vi "main_queue_assistant.vi"(0 "queue_type (def=all)":T3=enum."entities_incoming", 1 "action (enq_behind = def)":T8=enum."enq_behind", 2 "entity":T6, 3 "entities":T6[](array[typedef]), 4 "classpath / id (in)":string, 5 "error in (no error)":errorcluster, 6 "classpaths_for_queue_identification (ids)":string[](array[string]), 7 "timestep":dbl, 9 "response":T4) -> (15 "refs (out)":T1, 18 "queues_empty_status (out)":T2[](array[typedef]), 19 "error out":errorcluster)   [LabVIEW 2016]
uses:
  controls/queue_assistant_actions.ctl
  controls/entity.ctl
  controls/entity_type.ctl
  controls/queue_type.ctl
  controls/response.ctl
  controls/response_type.ctl
  controls/queue_status.ctl
  controls/queue_references.ctl
  controls/queue_assistant_runtime_object.ctl
panel:
  in  "queue out":refnum<queue>
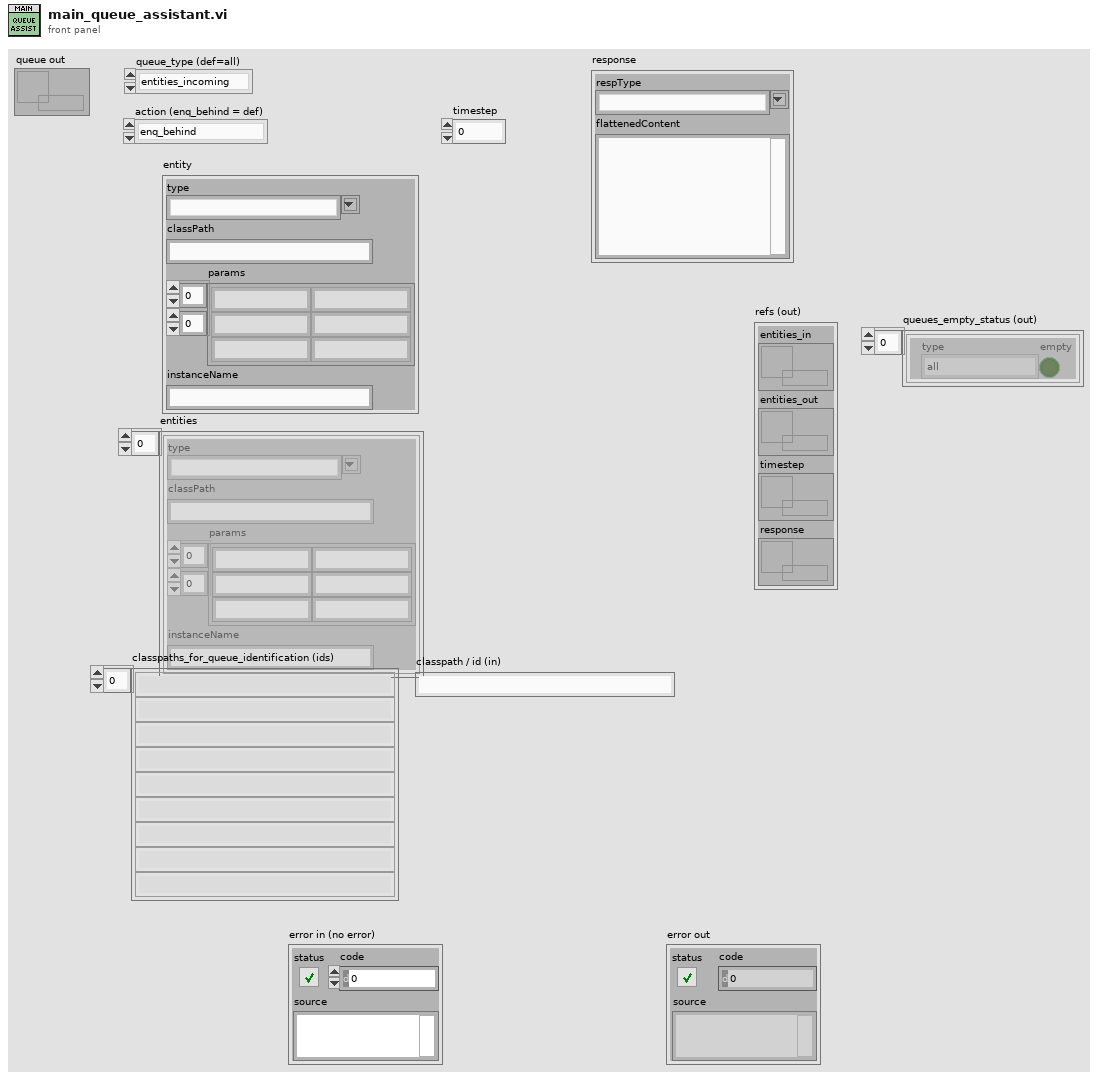
[diagram p1: front panel]
types:
  T1 = typedef "queue_references.ctl" = cluster{"entities_in":refnum<queue>, "entities_out":refnum<queue>, "timestep":refnum<queue>, "response":refnum<queue>}
  T2 = typedef "queue_status.ctl" = cluster{"type":T3, "empty":bool}
  T3 = typedef "queue_type.ctl" = enum16{"all", "dostep", "entities_incoming", "entities_outoing", "response"}
  T4 = typedef "response.ctl" = cluster{"respType":T5, "flattenedContent":string}
  T5 = typedef "response_type.ctl" = string
  T6 = typedef "entity.ctl" = cluster{"type":T7, "classPath":string, "params":string[][], "instanceName":string}
  T7 = typedef "entity_type.ctl" = string
  T8 = typedef "queue_assistant_actions.ctl" = enum16{"--- unused ---", "bulk_enq_ahead", "bulk_enq_behind", "destroy", "empty?", "enq_ahead", "enq_behind", "flush", "get_queues", "init"}
  T9 = typedef "queue_assistant_runtime_object.ctl" = cluster{"classpath":string, "queue":refnum<queue>}
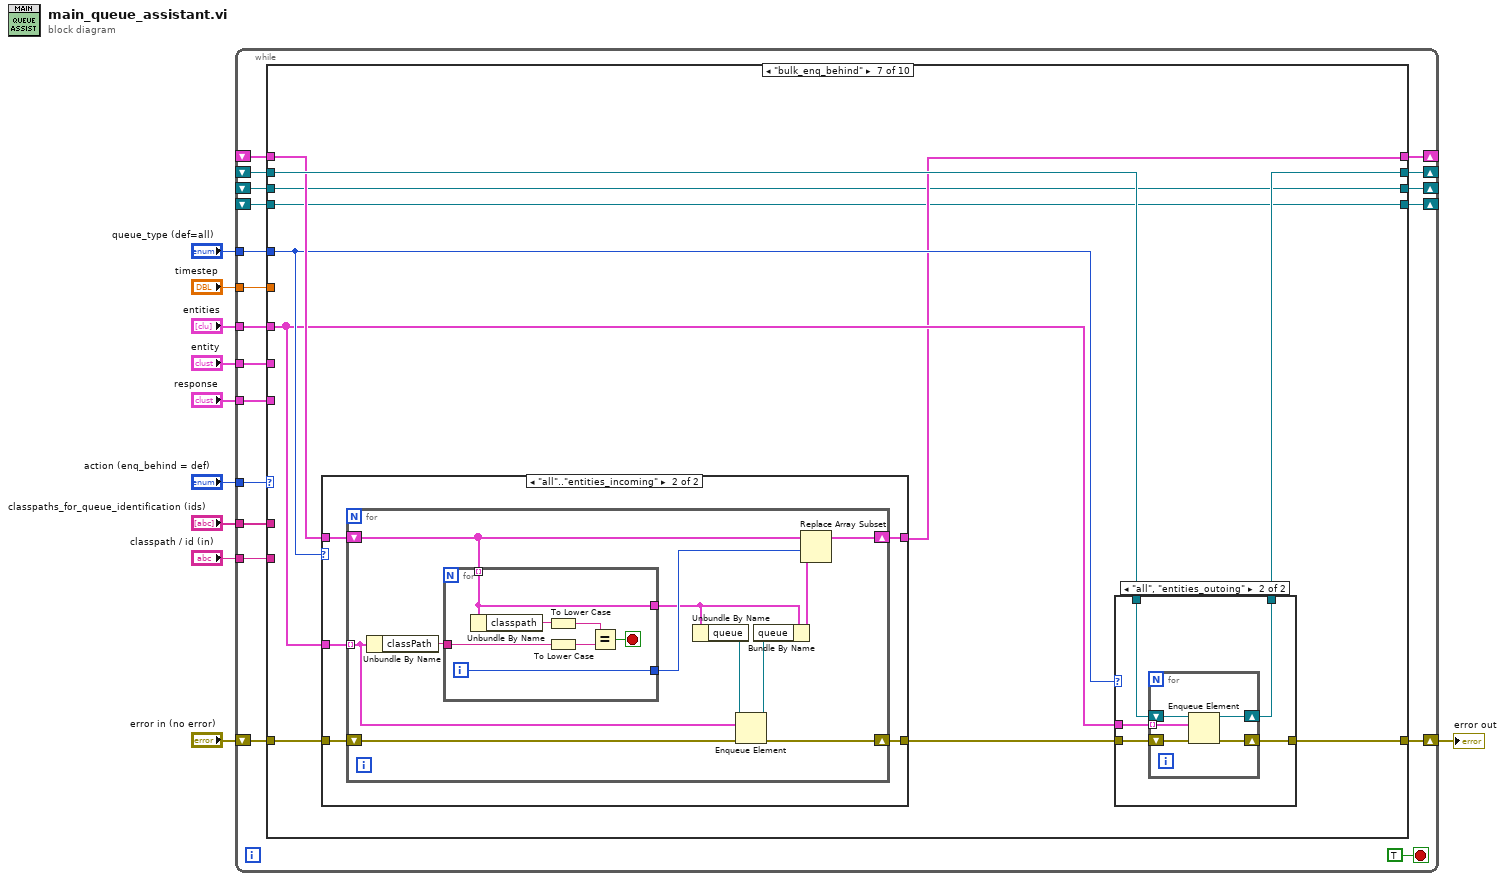
[diagram p0: block diagram]
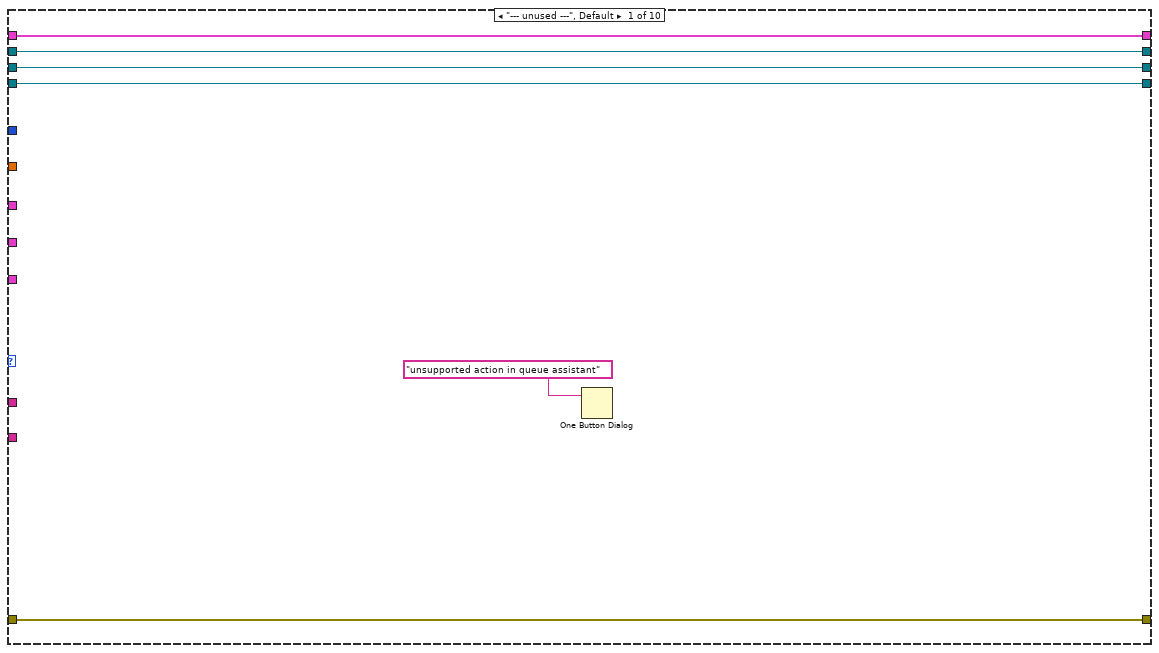
[diagram p2: hidden frame]
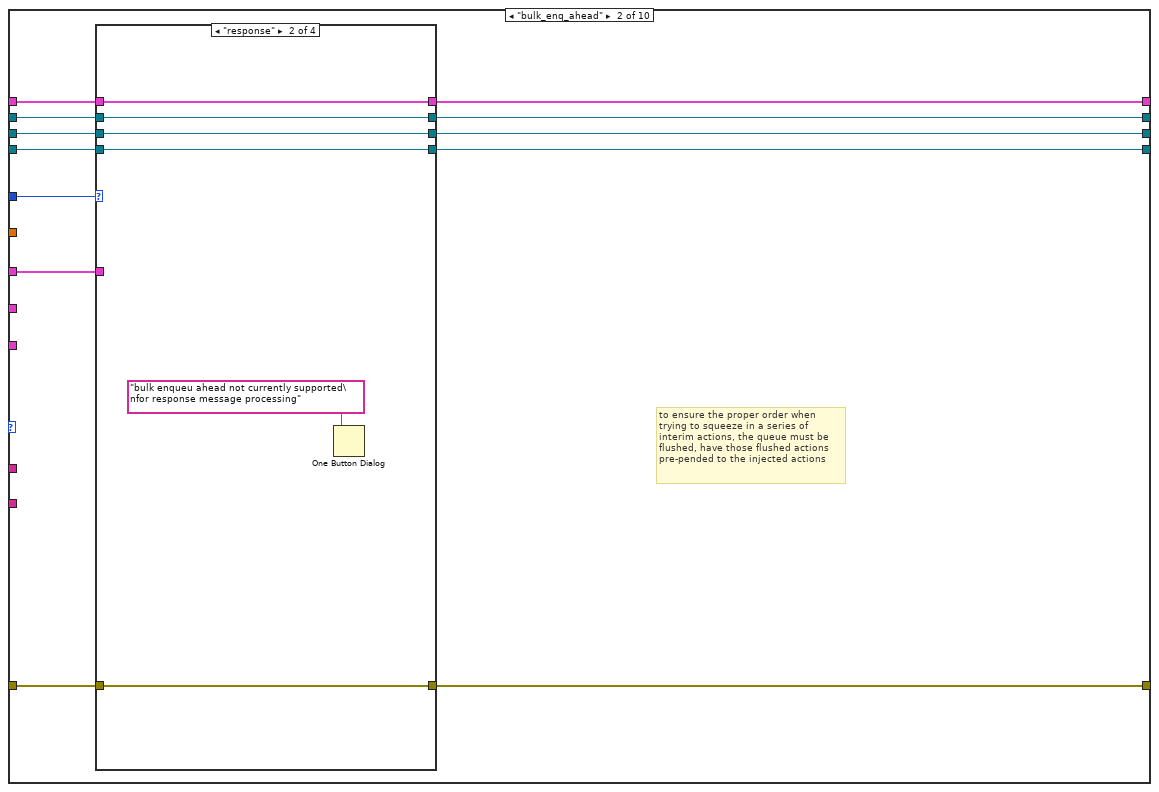
[diagram p3: hidden frame]
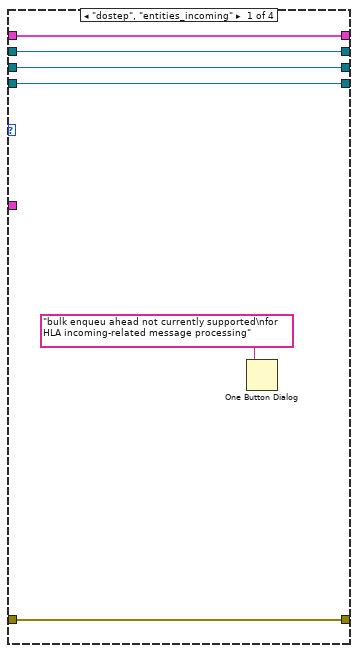
[diagram p4: hidden frame]
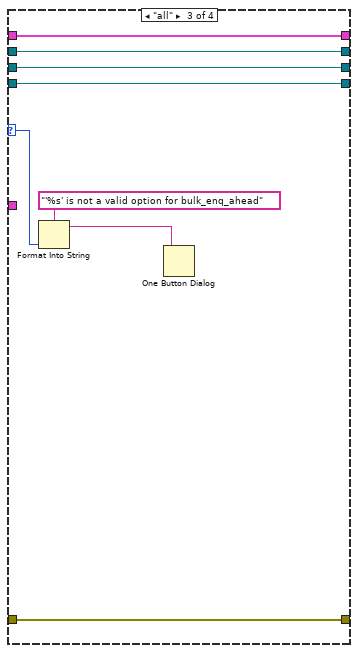
[diagram p5: hidden frame]
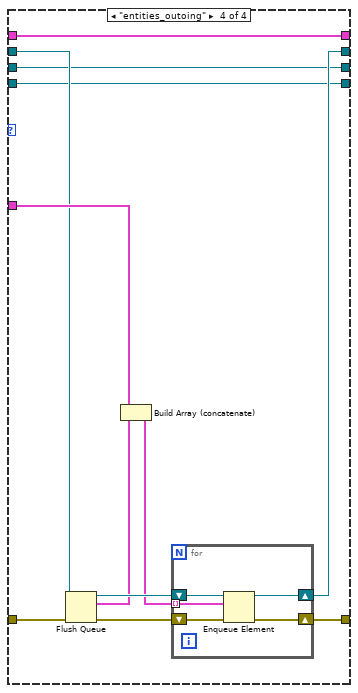
[diagram p6: hidden frame]
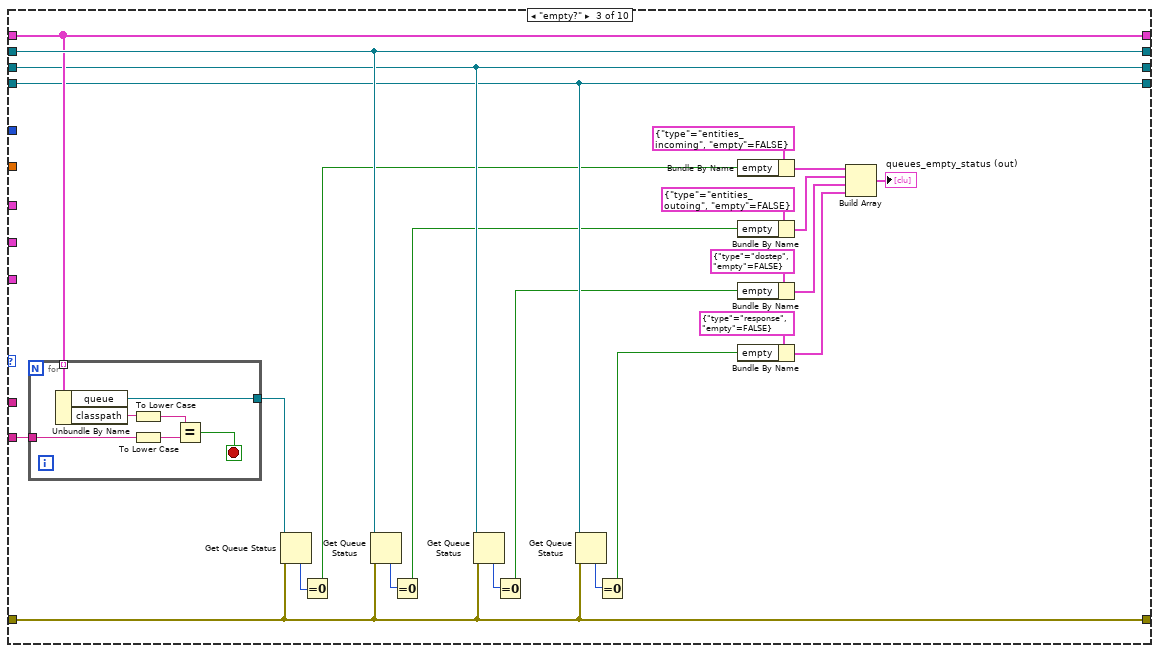
[diagram p7: hidden frame]
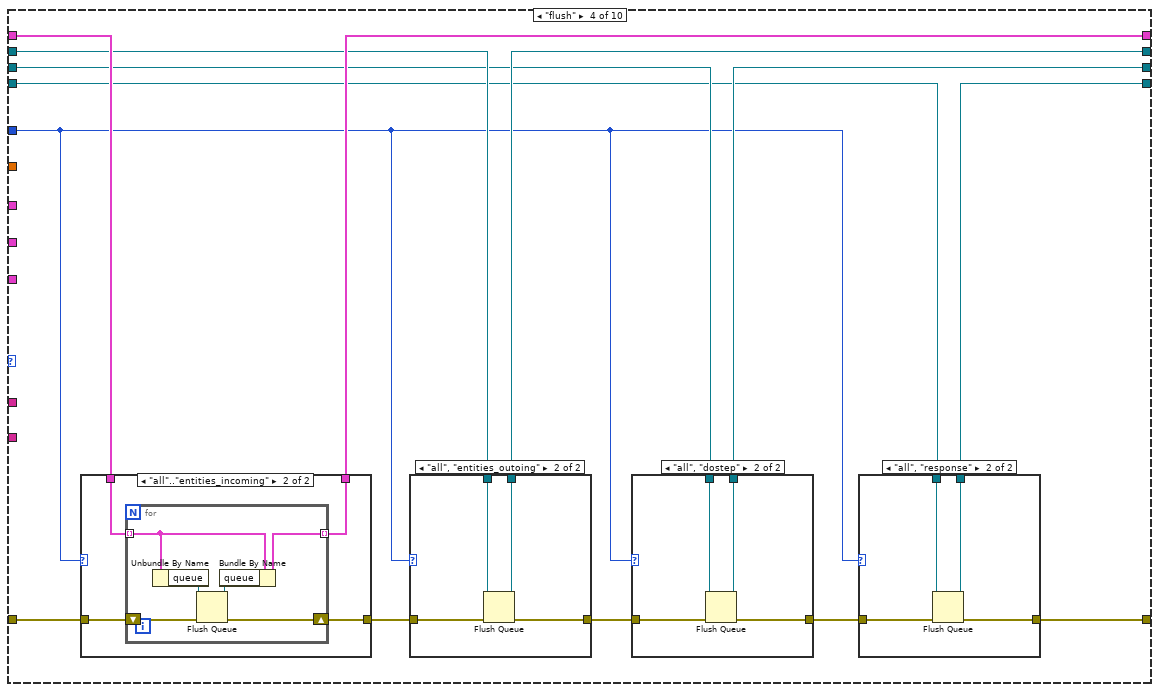
[diagram p8: hidden frame]
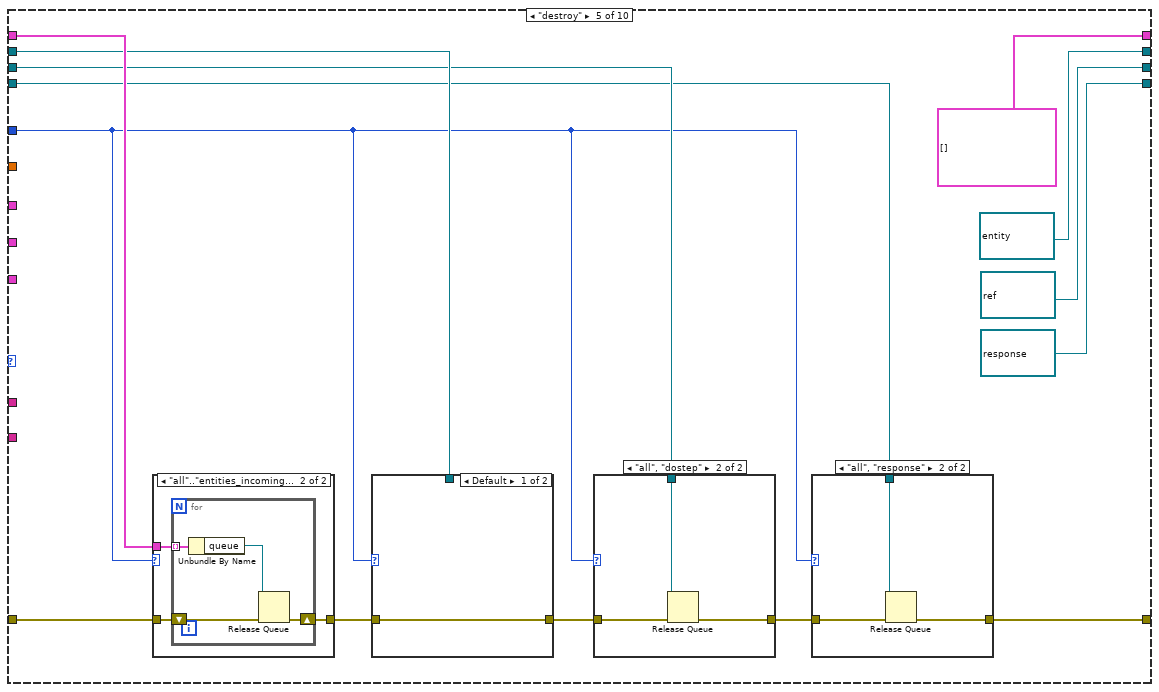
[diagram p13: hidden frame]
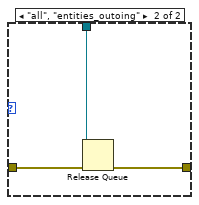
[diagram p16: hidden frame]
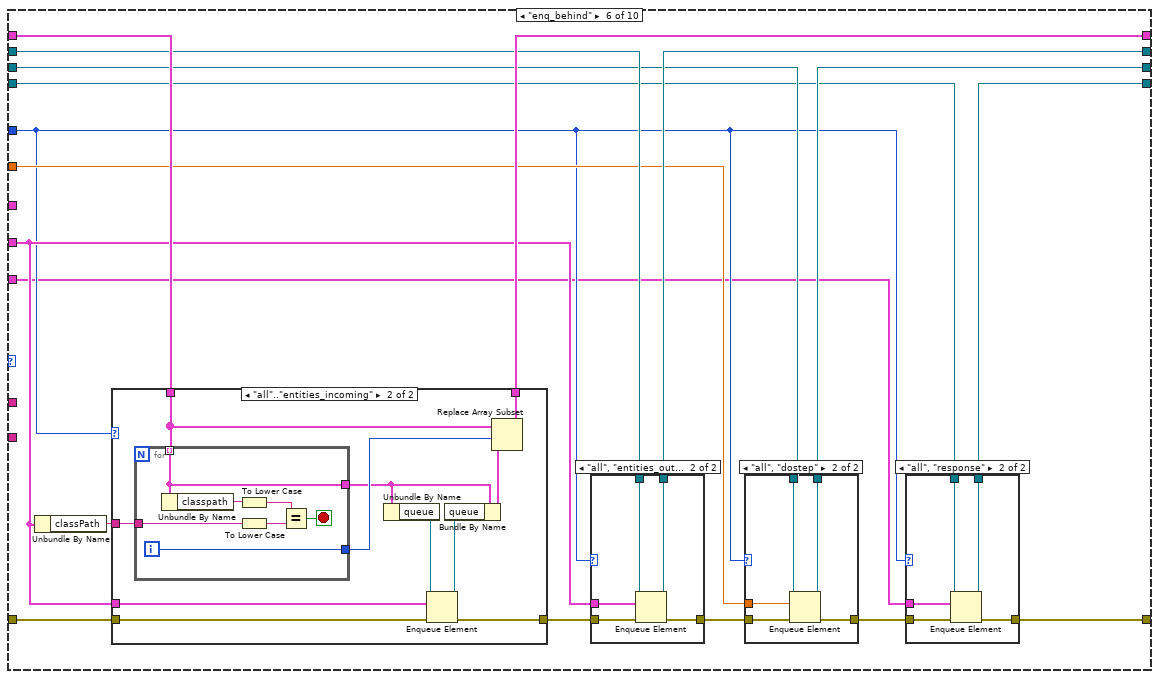
[diagram p18: hidden frame]
diagram:
  n1 = while {
    shift-right: [w22] -> _
    shift-left: _ -> [w25]
    tunnel: "action (enq_behind = def)" -> [w28]
    shift-right: [w26] -> w8
    shift-left: "error in (no error)" -> [w27]
    tunnel: "entity" -> [w24]
    tunnel: "entities" -> [w23]
    shift-right: [w21] -> _
    shift-left: _ -> [w20]
    tunnel: "queue_type (def=all)" -> [w19]
    tunnel: "classpaths_for_queue_identification (ids)" -> [w18]
    tunnel: "classpath / id (in)" -> [w17]
    shift-right: [w15] -> _
    shift-left: _ -> [w16]
    tunnel: "timestep" -> [w14]
    tunnel: "response" -> [w13]
    shift-right: [w12] -> _
    shift-left: _ -> [w11]
    stop <- TRUE stop-if-true
    n2 = case shown="\"bulk_enq_behind\"" w28 {
      tunnel: w27 -> [w34 w47 w85 w128 w173 w210 w257 w315 w366 w392]
      tunnel: [w34 w45 w85 w118 w160 w194 w263 w304 w366 w377] -> w26
      tunnel: w25 -> [w33 w46 w104 w129 w171 w211 w260 w313 w368 _]
      tunnel: w24 -> [_ _ _ _ _ w205 _ w314 _ _]
      tunnel: w23 -> [_ w44 _ _ _ _ w258 _ _ _]
      tunnel: [w33 w42 w104 w127 T9[] [] w209 w256 w312 w368 w391] -> w22
      tunnel: [w32 w40 w106 w124 refnum<queue> refnum ("queue out") w206 w261 w317 w362 w388] -> w21
      tunnel: w20 -> [w32 w41 w106 w125 w170 w207 w262 w318 w362 w389]
      tunnel: w19 -> [_ w43 _ w120 w163 w198 w259 w303 _ _]
      tunnel: w18 -> [_ _ _ _ _ _ _ _ _ w386]
      tunnel: w17 -> [_ _ w105 _ _ _ _ _ w369 _]
      tunnel: w16 -> [w31 w39 w101 w122 w167 w202 w254 w308 w363 w382]
      tunnel: [w31 w38 w101 w121 refnum<queue> refnum ("queue out") w201 w254 w307 w363 w383] -> w15
      tunnel: w14 -> [_ _ _ _ _ w200 _ w309 _ _]
      tunnel: w13 -> [_ _ _ _ _ w197 _ w305 _ _]
      tunnel: [w30 w36 w99 w116 refnum<queue> refnum ("queue out") w195 w253 w301 w364 w379] -> w12
      tunnel: w11 -> [w30 w37 w99 w117 w161 w196 w253 w302 w364 w378]
      frame "--- unused ---", Default {
        n3 = One Button Dialog(message="unsupported action in queue assistant") -> ()  [unwired: 1 in, 1 out]
      }
      frame "bulk_enq_ahead" {
        # "to ensure the proper order when\ntrying to squeeze in a series of\ninterim actions, the queue must be\nflushed, have those flushed actions\npre-pended to the injected actions"
        n4 = case shown="\"response\"" w43 {
          selector: w43 -> [_ _ w63 _]
          tunnel: w47 -> [w51 w57 w65 w79]
          tunnel: w46 -> [w53 w59 w67 w70]
          tunnel: [w51 w57 w65 w77] -> w45
          tunnel: w44 -> [_ _ _ w73]
          tunnel: [w53 w59 w67 w70] -> w42
          tunnel: w41 -> [w52 w58 w66 w72]
          tunnel: [w52 w58 w66 w71] -> w40
          tunnel: [w49 w55 w61 w69] -> w38
          tunnel: w39 -> [w49 w55 w61 w69]
          tunnel: [w48 w54 w60 w68] -> w36
          tunnel: w37 -> [w48 w54 w60 w68]
          frame "dostep", "entities_incoming" {
            n5 = One Button Dialog(message="bulk enqueu ahead not currently supported\nfor HLA incoming-related message processing") -> ()  [unwired: 1 in, 1 out]
          }
          frame "response" {
            n6 = One Button Dialog(message="bulk enqueu ahead not currently supported\nfor response message processing") -> ()  [unwired: 1 in, 1 out]
          }
          frame "all" {
            n7 = Format Into String(format string="'%s' is not a valid option for bulk_enq_ahead", w63) -> (resulting string=w62:string)  [unwired: 2 in, 1 out]
            n8 = One Button Dialog(message=w62) -> ()  [unwired: 1 in, 1 out]
          }
          frame "entities_outoing" {
            n9 = Flush Queue(queue=w72, error in (no error)=w79) -> (queue out=w76:refnum<queue>, remaining elements=w74:T6[], error out=w78:errorcluster)
            n10 = Build Array (concatenate)(w73, w74) -> (w75:T6[])
            n11 = for {
              shift-right: [w83] -> w77
              shift-left: w78 -> [w84]
              shift-right: [w81] -> w71
              shift-left: w76 -> [w82]
              tunnel: w75 -> [w80] mode=indexing
              n12 = Enqueue Element(queue=w82, element=w80, error in (no error)=w84) -> (queue out=w81:refnum<queue>, error out=w83:errorcluster)  [unwired: 1 in, 1 out]
            }
          }
        }
      }
      frame "empty?" {
        n13 = for {
          tunnel: w105 -> [w114]
          tunnel: w104 -> [w110] mode=indexing
          tunnel: [w109] -> w103
          stop <- w111 stop-if-true
          n14 = Unbundle By Name(w110) -> ("queue"=w109:refnum<queue>, "classpath"=w115:string)
          n15 = To Lower Case(string=w115) -> (all lower case string=w112:string)
          n16 = To Lower Case(string=w114) -> (all lower case string=w113:string)
          n17 = Equal?(x=w112, y=w113) -> (x = y?=w111:bool)
        }
        n18 = Get Queue Status(queue=w103, error in (no error)=w85) -> (# elements in queue=w108:i32)  [unwired: 1 in, 7 out]
        n19 = Equal To 0?(x=w108) -> (x = 0?=w93:bool)
        n20 = Get Queue Status(queue=w106, error in (no error)=w85) -> (# elements in queue=w107:i32)  [unwired: 1 in, 7 out]
        n21 = Equal To 0?(x=w107) -> (x = 0?=w91:bool)
        n22 = Get Queue Status(queue=w101, error in (no error)=w85) -> (# elements in queue=w102:i32)  [unwired: 1 in, 7 out]
        n23 = Equal To 0?(x=w102) -> (x = 0?=w97:bool)
        n24 = Get Queue Status(queue=w99, error in (no error)=w85) -> (# elements in queue=w100:i32)  [unwired: 1 in, 7 out]
        n25 = Equal To 0?(x=w100) -> (x = 0?=w95:bool)
        n26 = Bundle By Name(cluster=T2 {"type"=enum."entities_incoming", "empty"=FALSE} ("queue_status"), "empty"=w93) -> (w90:T2)
        n27 = Bundle By Name(cluster=T2 {"type"=enum."entities_outoing", "empty"=FALSE} ("queue_status"), "empty"=w91) -> (w89:T2)
        n28 = Bundle By Name(cluster=T2 {"type"=enum."dostep", "empty"=FALSE} ("queue_status"), "empty"=w97) -> (w88:T2)
        n29 = Bundle By Name(cluster=T2 {"type"=enum."response", "empty"=FALSE} ("queue_status"), "empty"=w95) -> (w87:T2)
        n30 = Build Array(w90, w89, w88, w87) -> (→"queues_empty_status (out)":T2[])
      }
      frame "flush" {
        n31 = case shown="\"all\"..\"entities_incoming\"" w120 {
          tunnel: [w149 w153] -> w126
          tunnel: w129 -> [w148 w152]
          tunnel: w128 -> [w149 w151]
          tunnel: [w148 w150] -> w127
          frame Default {
          }
          frame "all".."entities_incoming" {
            n32 = for {
              tunnel: w152 -> [w157] mode=indexing
              tunnel: [w156] -> w150 mode=indexing
              shift-right: [w159] -> w153
              shift-left: w151 -> [w158]
              n33 = Unbundle By Name(w157) -> ("queue"=w155:refnum<queue>)
              n34 = Flush Queue(queue=w155, error in (no error)=w158) -> (queue out=w154:refnum<queue>, error out=w159:errorcluster)  [unwired: 1 out]
              n35 = Bundle By Name(cluster=w157, "queue"=w154) -> (w156:T9)
            }
          }
        }
        n36 = case shown="\"all\", \"entities_outoing\"" w120 {
          tunnel: [w143 w147] -> w123
          tunnel: w125 -> [w142 w146]
          tunnel: w126 -> [w143 w145]
          tunnel: [w142 w144] -> w124
          frame Default {
          }
          frame "all", "entities_outoing" {
            n37 = Flush Queue(queue=w146, error in (no error)=w145) -> (queue out=w144:refnum<queue>, error out=w147:errorcluster)  [unwired: 1 out]
          }
        }
        n38 = case shown="\"all\", \"dostep\"" w120 {
          tunnel: [w137 w141] -> w119
          tunnel: w122 -> [w136 w140]
          tunnel: w123 -> [w137 w139]
          tunnel: [w136 w138] -> w121
          frame Default {
          }
          frame "all", "dostep" {
            n39 = Flush Queue(queue=w140, error in (no error)=w139) -> (queue out=w138:refnum<queue>, error out=w141:errorcluster)  [unwired: 1 out]
          }
        }
        n40 = case shown="\"all\", \"response\"" w120 {
          tunnel: [w131 w135] -> w118
          tunnel: w117 -> [w130 w134]
          tunnel: w119 -> [w131 w133]
          tunnel: [w130 w132] -> w116
          frame Default {
          }
          frame "all", "response" {
            n41 = Flush Queue(queue=w134, error in (no error)=w133) -> (queue out=w132:refnum<queue>, error out=w135:errorcluster)  [unwired: 1 out]
          }
        }
      }
      frame "destroy" {
        n42 = case shown="\"all\"..\"entities_incoming\"" w163 {
          tunnel: [w186 w189] -> w172
          tunnel: w171 -> [_ w187]
          tunnel: w173 -> [w186 w188]
          frame Default {
          }
          frame "all".."entities_incoming" {
            n43 = for {
              shift-right: [w193] -> w189
              shift-left: w188 -> [w192]
              tunnel: w187 -> [w191] mode=indexing
              n44 = Unbundle By Name(w191) -> ("queue"=w190:refnum<queue>)
              n45 = Release Queue(queue=w190, error in (no error)=w192) -> (error out=w193:errorcluster)  [unwired: 1 in, 2 out]
            }
          }
        }
        n46 = case shown="Default" w163 {
          tunnel: [w182 w185] -> w168
          tunnel: w170 -> [_ w184]
          tunnel: w172 -> [w182 w183]
          frame Default {
          }
          frame "all", "entities_outoing" {
            n47 = Release Queue(queue=w184, error in (no error)=w183) -> (error out=w185:errorcluster)  [unwired: 1 in, 2 out]
          }
        }
        n48 = case shown="\"all\", \"dostep\"" w163 {
          tunnel: [w178 w181] -> w162
          tunnel: w167 -> [_ w180]
          tunnel: w168 -> [w178 w179]
          frame Default {
          }
          frame "all", "dostep" {
            n49 = Release Queue(queue=w180, error in (no error)=w179) -> (error out=w181:errorcluster)  [unwired: 1 in, 2 out]
          }
        }
        n50 = case shown="\"all\", \"response\"" w163 {
          tunnel: [w174 w177] -> w160
          tunnel: w161 -> [_ w176]
          tunnel: w162 -> [w174 w175]
          frame Default {
          }
          frame "all", "response" {
            n51 = Release Queue(queue=w176, error in (no error)=w175) -> (error out=w177:errorcluster)  [unwired: 1 in, 2 out]
          }
        }
      }
      frame "enq_behind" {
        n52 = Unbundle By Name(w205) -> ("classPath"=w204:string)
        n53 = case shown="\"all\"..\"entities_incoming\"" w198 {
          tunnel: [w234 w245] -> w208
          tunnel: w211 -> [w233 w240]
          tunnel: w210 -> [w234 w244]
          tunnel: [w233 w239] -> w209
          tunnel: w205 -> [_ w235]
          tunnel: w204 -> [_ w243]
          frame Default {
          }
          frame "all".."entities_incoming" {
            n54 = for {
              tunnel: w243 -> [w251]
              tunnel: w240 -> [w246] mode=indexing
              tunnel: [w246] -> w238
              tunnel: [w247] -> w241
              i -> [w247]
              stop <- w248 stop-if-true
              n55 = Unbundle By Name(w246) -> ("classpath"=w252:string)
              n56 = To Lower Case(string=w252) -> (all lower case string=w249:string)
              n57 = To Lower Case(string=w251) -> (all lower case string=w250:string)
              n58 = Equal?(x=w249, y=w250) -> (x = y?=w248:bool)
            }
            n59 = Unbundle By Name(w238) -> ("queue"=w242:refnum<queue>)
            n60 = Enqueue Element(queue=w242, element=w235, error in (no error)=w244) -> (queue out=w237:refnum<queue>, error out=w245:errorcluster)  [unwired: 1 in, 1 out]
            n61 = Bundle By Name(cluster=w238, "queue"=w237) -> (w236:T9)
            n62 = Replace Array Subset(array=w240, new element=w236, index=w241) -> (w239:T9[])
          }
        }
        n63 = case shown="\"all\", \"entities_outoing\"" w198 {
          tunnel: [w227 w232] -> w203
          tunnel: w207 -> [w226 w231]
          tunnel: w208 -> [w227 w230]
          tunnel: [w226 w229] -> w206
          tunnel: w205 -> [_ w228]
          frame Default {
          }
          frame "all", "entities_outoing" {
            n64 = Enqueue Element(queue=w231, element=w228, error in (no error)=w230) -> (queue out=w229:refnum<queue>, error out=w232:errorcluster)  [unwired: 1 in, 1 out]
          }
        }
        n65 = case shown="\"all\", \"dostep\"" w198 {
          tunnel: [w220 w225] -> w199
          tunnel: w202 -> [w219 w224]
          tunnel: w203 -> [w220 w223]
          tunnel: [w219 w222] -> w201
          tunnel: w200 -> [_ w221]
          frame Default {
          }
          frame "all", "dostep" {
            n66 = Enqueue Element(queue=w224, element=w221, error in (no error)=w223) -> (queue out=w222:refnum<queue>, error out=w225:errorcluster)  [unwired: 1 in, 1 out]
          }
        }
        n67 = case shown="\"all\", \"response\"" w198 {
          tunnel: [w213 w218] -> w194
          tunnel: w196 -> [w212 w217]
          tunnel: w199 -> [w213 w216]
          tunnel: [w212 w215] -> w195
          tunnel: w197 -> [_ w214]
          frame Default {
          }
          frame "all", "response" {
            n68 = Enqueue Element(queue=w217, element=w214, error in (no error)=w216) -> (queue out=w215:refnum<queue>, error out=w218:errorcluster)  [unwired: 1 in, 1 out]
          }
        }
      }
      frame "bulk_enq_behind" {
        n69 = case shown="\"all\"..\"entities_incoming\"" w259 {
          tunnel: [w265 w270] -> w255
          tunnel: w257 -> [w265 w269]
          tunnel: w258 -> [_ w268]
          tunnel: w260 -> [w264 w267]
          tunnel: [w264 w266] -> w256
          frame Default {
          }
          frame "all".."entities_incoming" {
            n70 = for {
              tunnel: w268 -> [w271] mode=indexing
              shift-right: [w273] -> w266
              shift-left: w267 -> [w274]
              shift-right: [w281] -> w270
              shift-left: w269 -> [w280]
              n71 = Unbundle By Name(w271) -> ("classPath"=w272:string)
              n72 = for {
                tunnel: w272 -> [w287]
                tunnel: w274 -> [w282] mode=indexing
                tunnel: [w282] -> w277
                tunnel: [w283] -> w278
                i -> [w283]
                stop <- w284 stop-if-true
                n73 = Unbundle By Name(w282) -> ("classpath"=w288:string)
                n74 = To Lower Case(string=w288) -> (all lower case string=w285:string)
                n75 = To Lower Case(string=w287) -> (all lower case string=w286:string)
                n76 = Equal?(x=w285, y=w286) -> (x = y?=w284:bool)
              }
              n77 = Unbundle By Name(w277) -> ("queue"=w279:refnum<queue>)
              n78 = Enqueue Element(queue=w279, element=w271, error in (no error)=w280) -> (queue out=w276:refnum<queue>, error out=w281:errorcluster)  [unwired: 1 in, 1 out]
              n79 = Bundle By Name(cluster=w277, "queue"=w276) -> (w275:T9)
              n80 = Replace Array Subset(array=w274, new element=w275, index=w278) -> (w273:T9[])
            }
          }
        }
        n81 = case shown="\"all\", \"entities_outoing\"" w259 {
          tunnel: [w290 w294] -> w263
          tunnel: w262 -> [w289 w293]
          tunnel: w255 -> [w290 w295]
          tunnel: [w289 w291] -> w261
          tunnel: w258 -> [_ w292]
          frame Default {
          }
          frame "all", "entities_outoing" {
            n82 = for {
              shift-right: [w299] -> w294
              shift-left: w295 -> [w300]
              shift-right: [w297] -> w291
              shift-left: w293 -> [w298]
              tunnel: w292 -> [w296] mode=indexing
              n83 = Enqueue Element(queue=w298, element=w296, error in (no error)=w300) -> (queue out=w297:refnum<queue>, error out=w299:errorcluster)  [unwired: 1 in, 1 out]
            }
          }
        }
      }
      frame "enq_ahead" {
        n84 = Unbundle By Name(w314) -> ("classPath"=w316:string)
        n85 = case shown="\"all\"..\"entities_incoming\"" w303 {
          tunnel: [w334 w345] -> w311
          tunnel: w313 -> [w333 w340]
          tunnel: w315 -> [w334 w344]
          tunnel: [w333 w339] -> w312
          tunnel: w314 -> [_ w335]
          tunnel: w316 -> [_ w343]
          frame Default {
          }
          frame "all".."entities_incoming" {
            n86 = for {
              tunnel: w343 -> [w351]
              tunnel: w340 -> [w346] mode=indexing
              tunnel: [w346] -> w338
              tunnel: [w347] -> w341
              i -> [w347]
              stop <- w348 stop-if-true
              n87 = Unbundle By Name(w346) -> ("classpath"=w352:string)
              n88 = To Lower Case(string=w352) -> (all lower case string=w349:string)
              n89 = To Lower Case(string=w351) -> (all lower case string=w350:string)
              n90 = Equal?(x=w349, y=w350) -> (x = y?=w348:bool)
            }
            n91 = Unbundle By Name(w338) -> ("queue"=w342:refnum<queue>)
            n92 = Enqueue Element(queue=w342, element=w335, error in (no error)=w344) -> (queue out=w337:refnum<queue>, error out=w345:errorcluster)  [unwired: 1 in, 1 out]
            n93 = Bundle By Name(cluster=w338, "queue"=w337) -> (w336:T9)
            n94 = Replace Array Subset(array=w340, new element=w336, index=w341) -> (w339:T9[])
          }
        }
        n95 = case shown="\"all\", \"entities_outoing\"" w303 {
          tunnel: [w354 w359] -> w310
          tunnel: w318 -> [w353 w358]
          tunnel: w311 -> [w354 w357]
          tunnel: [w353 w356] -> w317
          tunnel: w314 -> [_ w355]
          frame Default {
          }
          frame "all", "entities_outoing" {
            n96 = Enqueue Element At Opposite End(queue=w358, element=w355, error in (no error)=w357) -> (queue out=w356:refnum<queue>, error out=w359:errorcluster)  [unwired: 1 in, 1 out]
          }
        }
        n97 = case shown="\"all\", \"dostep\"" w303 {
          tunnel: [w327 w332] -> w306
          tunnel: w308 -> [w326 w331]
          tunnel: w310 -> [w327 w330]
          tunnel: [w326 w329] -> w307
          tunnel: w309 -> [_ w328]
          frame Default {
          }
          frame "all", "dostep" {
            n98 = Enqueue Element At Opposite End(queue=w331, element=w328, error in (no error)=w330) -> (queue out=w329:refnum<queue>, error out=w332:errorcluster)  [unwired: 1 in, 1 out]
          }
        }
        n99 = case shown="\"all\", \"response\"" w303 {
          tunnel: [w320 w325] -> w304
          tunnel: w302 -> [w319 w324]
          tunnel: w306 -> [w320 w323]
          tunnel: [w319 w322] -> w301
          tunnel: w305 -> [_ w321]
          frame Default {
          }
          frame "all", "response" {
            n100 = Enqueue Element At Opposite End(queue=w324, element=w321, error in (no error)=w323) -> (queue out=w322:refnum<queue>, error out=w325:errorcluster)  [unwired: 1 in, 1 out]
          }
        }
      }
      frame "get_queues" {
        n101 = for {
          tunnel: w369 -> [w375]
          tunnel: w368 -> [w370] mode=indexing
          tunnel: [w370] -> w367
          tunnel: [w371] -> _
          i -> [w371]
          stop <- w372 stop-if-true
          n102 = Unbundle By Name(w370) -> ("classpath"=w376:string)
          n103 = To Lower Case(string=w376) -> (all lower case string=w373:string)
          n104 = To Lower Case(string=w375) -> (all lower case string=w374:string)
          n105 = Equal?(x=w373, y=w374) -> (x = y?=w372:bool)
        }
        n106 = Unbundle By Name(w367) -> ("queue"=w361:refnum<queue>)
        n107 = Bundle By Name(cluster=T1 {"entities_in"=refnum, "entities_out"=refnum, "timestep"=refnum, "response"=refnum} ("refs (out)"), "response"=w364, "timestep"=w363, "entities_out"=w362, "entities_in"=w361) -> (→"refs (out)":T1)
      }
      frame "init" {
        # "initialize a series of queues, one for each interaction/object\noriginally identified from the FOM file"
        n108 = for {
          tunnel: [w411] -> w391 mode=indexing
          shift-right: [w419] -> w387
          shift-left: w392 -> [w420]
          tunnel: w386 -> [w412] mode=indexing
          n109 = Format Into String(format string="%s_%s", queue_type."entities_incoming" ("queue_type"), w412) -> (resulting string=w417:string)  [unwired: 2 in, 1 out]
          n110 = Obtain Queue(name (unnamed)=w417, element data type=T6 {"type"="", "classPath"="", "params"=[], "instanceName"=""} ("entity"), error in (no error)=w420) -> (queue out=w413:refnum<queue>, error out=w419:errorcluster)  [unwired: 2 in, 1 out]
          n111 = Bundle By Name(cluster=T9 {"classpath"="", "queue"=refnum} ("queue_obj"), "classpath"=w412, "queue"=w413) -> (w411:T9)
        }
        n112 = Not A Number/Path/Refnum?(number/path/refnum=w389) -> (NaN/Path/Refnum?=w390:bool)
        n113 = case shown="True" w390 {
          tunnel: w387 -> [w421 w429]
          tunnel: [w422 w426] -> w388
          tunnel: w389 -> [w422 _]
          tunnel: [w421 w425] -> w384
          frame False {
          }
          frame True {
            n114 = Format Into String(format string="%s", queue_type."entities_outoing" ("queue_type")) -> (resulting string=w427:string)  [unwired: 2 in, 1 out]
            n115 = Obtain Queue(name (unnamed)=w427, element data type=T6 {"type"="", "classPath"="", "params"=[], "instanceName"=""} ("entity"), error in (no error)=w429) -> (queue out=w426:refnum<queue>, error out=w425:errorcluster)  [unwired: 2 in, 1 out]
          }
        }
        n116 = Not A Number/Path/Refnum?(number/path/refnum=w382) -> (NaN/Path/Refnum?=w385:bool)
        n117 = case shown="True" w385 {
          tunnel: w384 -> [w402 w410]
          tunnel: [w403 w407] -> w383
          tunnel: w382 -> [w403 _]
          tunnel: [w402 w406] -> w380
          frame False {
          }
          frame True {
            n118 = Format Into String(format string="%s", queue_type."dostep" ("queue_type")) -> (resulting string=w408:string)  [unwired: 2 in, 1 out]
            n119 = Obtain Queue(name (unnamed)=w408, element data type=0.0, error in (no error)=w410) -> (queue out=w407:refnum<queue>, error out=w406:errorcluster)  [unwired: 2 in, 1 out]
          }
        }
        n120 = Not A Number/Path/Refnum?(number/path/refnum=w378) -> (NaN/Path/Refnum?=w381:bool)
        n121 = case shown="True" w381 {
          tunnel: w380 -> [w393 w401]
          tunnel: [w394 w398] -> w379
          tunnel: w378 -> [w394 _]
          tunnel: [w393 w397] -> w377
          frame False {
          }
          frame True {
            n122 = Format Into String(format string="%s", queue_type."response" ("queue_type")) -> (resulting string=w399:string)  [unwired: 2 in, 1 out]
            n123 = Obtain Queue(name (unnamed)=w399, element data type=T4 {"respType"="", "flattenedContent"=""} ("response"), error in (no error)=w401) -> (queue out=w398:refnum<queue>, error out=w397:errorcluster)  [unwired: 2 in, 1 out]
          }
        }
      }
    }
  }
  "error out" <- w8
